vi "dynamics.vi"(8 "Control Input":dbl, 11 "State":T1) -> (3 "Future State":cluster{"Position":dbl, "Velocity":dbl})   [LabVIEW 2018]
uses:
  State.ctl
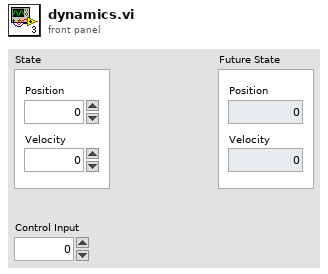
[diagram p1: front panel]
types:
  T1 = typedef "State.ctl" = cluster{"Position":dbl, "Velocity":dbl}
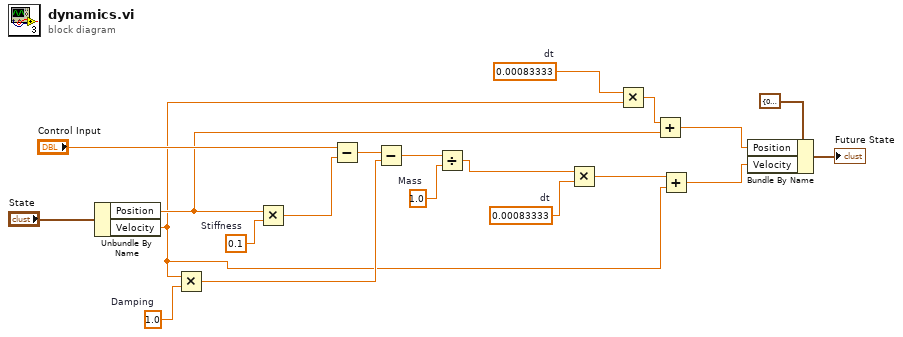
[diagram p0: block diagram]
diagram:
  w2 = 0.00083333  # dt
  w10 = 0.00083333  # dt
  w13 = 1.0  # Mass
  w18 = 1.0  # Damping
  w19 = 0.1  # Stiffness
  n1 = Unbundle By Name("State") -> ("Position"=w6:dbl, "Velocity"=w5:dbl)
  n2 = Multiply(x=w5, y=w18) -> (x*y=w9:dbl)
  n3 = Multiply(x=w6, y=w19) -> (x*y=w16:dbl)
  n4 = Subtract(x="Control Input", y=w16) -> (x-y=w15:dbl)
  n5 = Subtract(x=w15, y=w9) -> (x-y=w14:dbl)
  n6 = Divide(x=w14, y=w13) -> (x/y=w3:dbl)
  n7 = Multiply(x=w3, y=w2) -> (x*y=w1:dbl)
  n8 = Multiply(x=w10, y=w5) -> (x*y=w8:dbl)
  n9 = Add(x=w8, y=w6) -> (x+y=w7:dbl)
  n10 = Add(x=w1, y=w5) -> (x+y=w4:dbl)
  n11 = Bundle By Name(cluster=cluster{"Position":dbl, "Velocity":dbl} {"Position"=0.0, "Velocity"=0.0} ("State 2"), "Position"=w7, "Velocity"=w4) -> (→"Future State":cluster{"Position":dbl, "Velocity":dbl})
